vi "pc_half_height.vi"(8 "error in (no error)":errorcluster, 10 "y-data in":dbl[](array[numeric])) -> (0 "error out":errorcluster, 1 "half height out":dbl, 2 "y-data out":dbl[](array[numeric]))   [LabVIEW 2017, in "Plots.lvclass"]
doc: "computes the \"half heigt\" of the input data (usually y-data)"
uses:
  Plots.lvclass
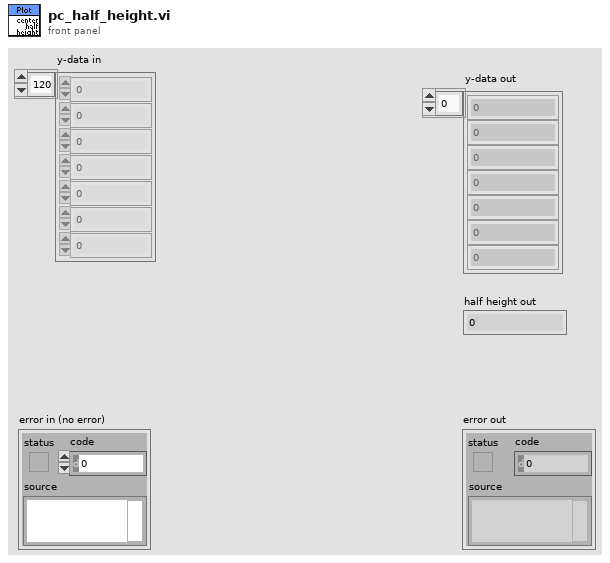
[diagram p1: front panel]
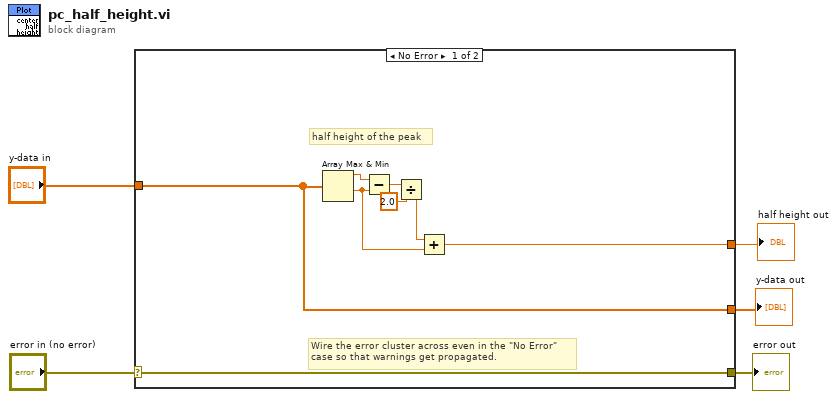
[diagram p0: block diagram]
diagram:
  n1 = case shown="No Error" "error in (no error)" {
    selector: "error in (no error)" -> [w13 w14]
    tunnel: [w13 w14] -> w4
    tunnel: "y-data in" -> [w6 _]
    tunnel: [w7 _] -> w2
    tunnel: [w6 _] -> w1
    frame No Error {
      # "half height of the peak"
      # "Wire the error cluster across even in the \"No Error\"\ncase so that warnings get propagated."
      n2 = Array Max & Min(array=w6) -> (max value=w10:dbl, min value=w8:dbl)  [unwired: 2 out]
      n3 = Subtract(x=w10, y=w8) -> (x-y=w11:dbl)
      n4 = Divide(x=w11, y=2.0) -> (x/y=w9:dbl)
      n5 = Add(x=w9, y=w8) -> (x+y=w7:dbl)
    }
    frame Error {
    }
  }
  "error out" <- w4
  "half height out" <- w2
  "y-data out" <- w1
